vi "Destroy User Event - Stop.vi"(8 "error in (no error)":errorcluster {"code" format="Error %.0f"}, 11 "userEvents":T1) -> (0 "error out":errorcluster {"code" format="Error %.0f"})   [LabVIEW 2017, in "User Event - Stop.lvlib"]
doc: "Destroy the user event, even if there is an incoming error."
uses:
  User Event - Stop.lvlib
  userEvents.ctl
  Controls/objectRefsMain.ctl
  sendRefs.ctl
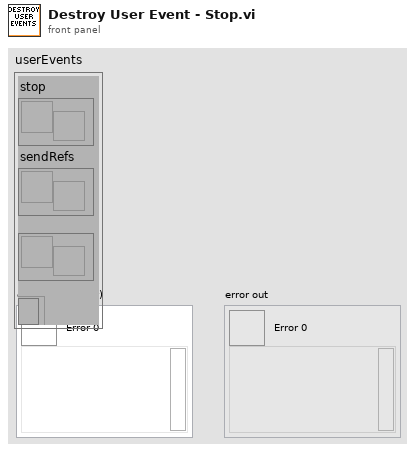
[diagram p1: front panel]
types:
  T1 = typedef "User Event - Stop.lvlib/userEvents.ctl" = cluster{"stop":refnum<user-event>, "sendRefs":refnum<user-event>, "sendSubVIRefs":refnum<user-event>, "eventRegRef":refnum<event-registration>}
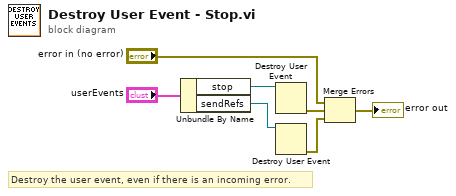
[diagram p0: block diagram]
diagram:
  # "Destroy the user event, even if there is an incoming error."
  n1 = Unbundle By Name("userEvents") -> ("stop"=w2:refnum<user-event>, "sendRefs"=w1:refnum<user-event>)
  n2 = Destroy User Event(user event=w2) -> (error out=w7:errorcluster)  [unwired: 1 in]
  n3 = Destroy User Event(user event=w1) -> (error out=w6:errorcluster)  [unwired: 1 in]
  n4 = Merge Errors("error in (no error)", w7, w6) -> (→"error out":errorcluster)
